vi "gRPC.Response.GetError.vi"(8 "error in (no error)":errorcluster, 11 "Response":variant) -> (0 "error out":errorcluster)   [LabVIEW 2025, in "XNET Bus Monitor Client.lvlib"]
uses:
  XNET Bus Monitor Client.lvlib
  bus_monitor_client/RPC Messages/ni_bus_monitor_api_ErrorInfo.ctl
  <userlib>/_OpenG.lib/lvdata/lvdata.llb/openg_variant.lvlib
  bus_monitor_client/bus_monitor_client.lvlib
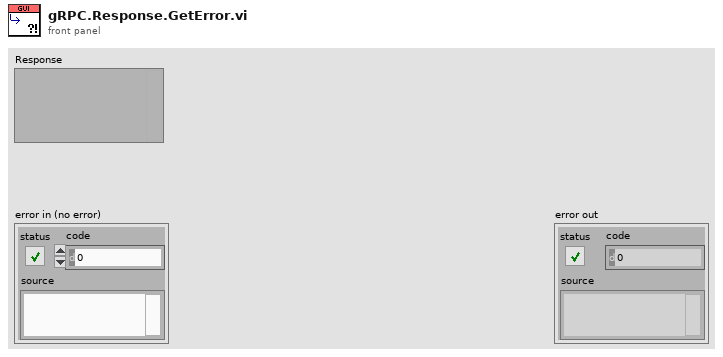
[diagram p1: front panel]
types:
  T1 = typedef "bus_monitor_client.lvlib/ni_bus_monitor_api_ErrorInfo.ctl" = errorcluster
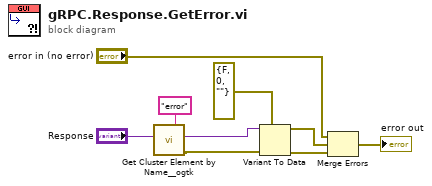
[diagram p0: block diagram]
diagram:
  n1 = call <userlib>:"Get Cluster Element by Name__ogtk.vi"("Element Name"="error", "Cluster"="Response") -> ("error out"=w7:errorcluster, "VElement"=w6:variant)  [unwired: 7 in, 1 out]
  n2 = Variant To Data(error in=w7, type=T1 {"status"=FALSE, "code"=0, "source"=""} ("error"), Variant=w6) -> (data=w1:T1, error out=w9:errorcluster)
  n3 = Merge Errors("error in (no error)", w1, w9) -> (→"error out":errorcluster)
